vi "PH_Beamline_Chief.set i attribute.vi"(0 "i ref in":refnum<vi>, 2 "i attribute":T1={"BL Service IDs"={"YLF_BL_Status"=-1, "fs_BL_Status"=-1, "fs_YLF_BL_Status"=-1, "ns_BL_Status"=-1, "PA_Input_BL_Status"=-1, "PA_UnDelay_BL_Status"=-1, "PA_Delay_BL_Status"=-1, "PA_BL_Status"=-1, "PA_Bypass_BL_Status"=-1, "PA_Exit_BL_Status"=-1, "PA_LL_BL_Status"=-1, "LL_BL_Status"=-1, "PA_MA_BL_Status"=-1, "MA_Exit_BL_Status"=-1, "MA_Z6_BL_Status"=-1, "Z6_BL_Status"=-1, "MA_LB_BL_Status"=-1, "LB_TB2_BL_Status"=-1, "PA_before_Bypass_BL_Status"=-1, "LB_TB3_BL_Status"=-1}, "R2S Service ID"=-1, "Settings"={"Wanted"={"PA Doublepass Mode"=FALSE, "Compressor Vaccuum LB not relevant"=FALSE, "Windowshutter TB2 not relevant"=FALSE, "Windowshutter TB3 not relevant"=FALSE}, "GUI Ref"=refnum, "Service ID"=-1}}, 5 "error in (no error)":errorcluster) -> (14 "i ref out":refnum<vi>, 19 "error out":errorcluster)   [LabVIEW 2014, in "PH_Beamline_Chief.lvlib"]
doc: "Sets the i attribute data of an object.\n\nLicense Agreement for this software:\n\nCopyright (C)\nGesellschaft für Schwerionenforschung, GSI\nPlanckstr. 1\n64291 Darmstadt\nGermany\n\nContact: D.Beck@gsi.de \n\nThis program is free software; you can redistribute it and/or modify it under the terms of the GNU General Public License as published by the Free Software Foundation; either version 2 of the license, or (at your option) any later version.\n\nThis program is distributed in the hope that it will be useful, but WITHOUT ANY WARRANTY; without even the implied warranty of MERCHANTABILITY or FITNESS FOR A PARTICULAR PURPOSE. See the GNU General License for more details (http://www.gnu.org).\n\nGesellschaft für Schwerionenforschung, GSI\nPlanckstr. 1, 64291 Darmstadt, Germany\nFor all questions and ideas contact: M.Richter@gsi.de, H.Brand@gsi.de or D.Beck@gsi.de.\nLast update: 17-JUN-2004"
uses:
  PH_Beamline_Chief.lvlib
  PH_Beamline_Chief.i attribute.ctl
  PH_Beamline_Chief.Settings.ctl
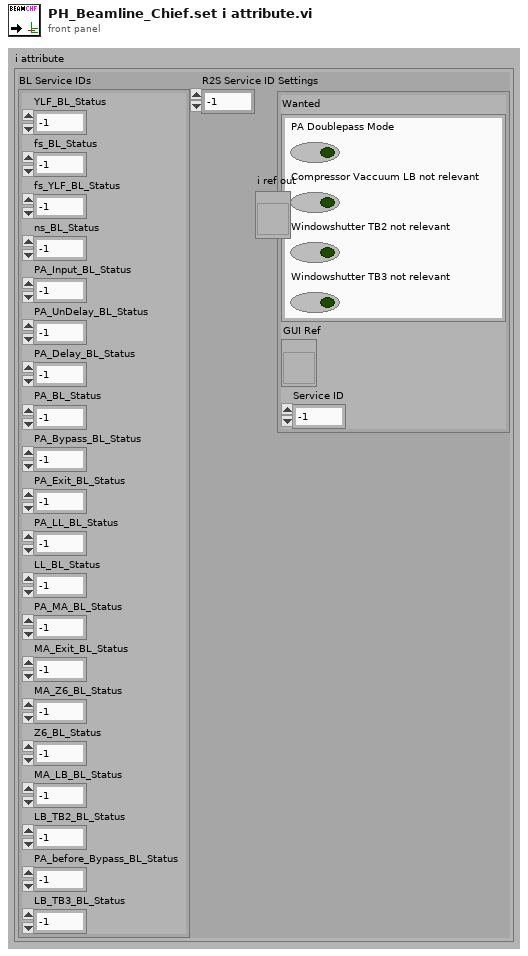
[diagram p1: front panel]
types:
  T1 = typedef "PH_Beamline_Chief.lvlib/PH_Beamline_Chief.i attribute.ctl" = cluster{"BL Service IDs":cluster{"YLF_BL_Status":i32, "fs_BL_Status":i32, "fs_YLF_BL_Status":i32, "ns_BL_Status":i32, "PA_Input_BL_Status":i32, "PA_UnDelay_BL_Status":i32, "PA_Delay_BL_Status":i32, "PA_BL_Status":i32, "PA_Bypass_BL_Status":i32, "PA_Exit_BL_Status":i32, "PA_LL_BL_Status":i32, "LL_BL_Status":i32, "PA_MA_BL_Status":i32, "MA_Exit_BL_Status":i32, "MA_Z6_BL_Status":i32, "Z6_BL_Status":i32, "MA_LB_BL_Status":i32, "LB_TB2_BL_Status":i32, "PA_before_Bypass_BL_Status":i32, "LB_TB3_BL_Status":i32}, "R2S Service ID":i32, "Settings":cluster{"Wanted":T2, "GUI Ref":refnum<vi>, "Service ID":i32}}
  T2 = typedef "PH_Beamline_Chief.lvlib/PH_Beamline_Chief.Settings.ctl" = cluster{"PA Doublepass Mode":bool, "Compressor Vaccuum LB not relevant":bool, "Windowshutter TB2 not relevant":bool, "Windowshutter TB3 not relevant":bool}
  T3 = enum16{"SetAttribute", "GetAttribute", "CreateAttribute", "DestroyAttribute", "DestroyAllAtributes"}
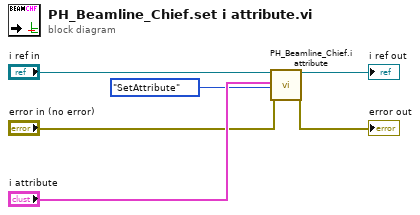
[diagram p0: block diagram]
diagram:
  n1 = call "PH_Beamline_Chief.i attribute.vi"("VI Refnum"="i ref in", "CLASS.i attribute"="i attribute", "Action"=T3."SetAttribute", "error in (no error)"="error in (no error)") -> ("VI Refnum out"=→"i ref out":refnum<vi>, "error out"=→"error out":errorcluster)  [unwired: 13 in, 1 out]
